vi "WVD Calculation.vi"(1 "time increment":i32, 2 "H[s]":dbl[](array[numeric]) format="%.2f", 3 "s":dbl[](array[numeric]) format="%.2f") -> (0 "Fourier[s(i-m)*g(m)]":sgl[][](array[numeric]) format="%.2f")   [LabVIEW 2017, in "NI_Gmath.lvlib"]
uses:
  <vilib>/gmath/NI_Gmath.lvlib
  <vilib>/Analysis/2dsp.llb/Complex FFT.vi
  <vilib>/Analysis/NI_AALPro.lvlib
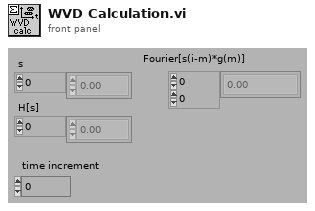
[diagram p1: front panel]
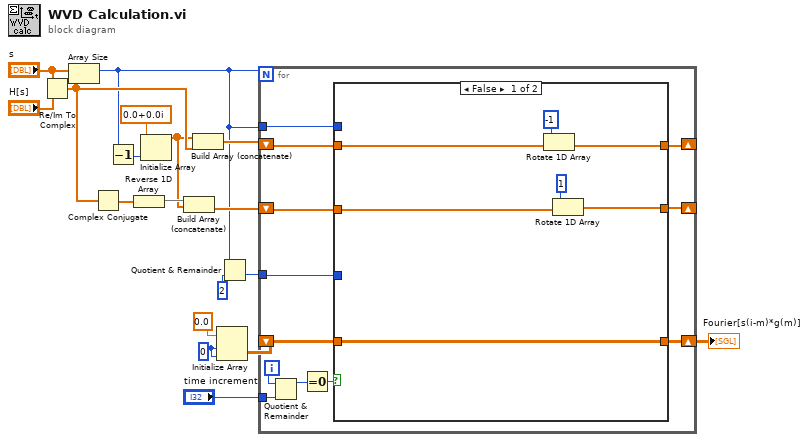
[diagram p0: block diagram]
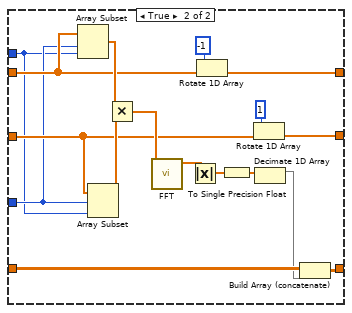
[diagram p2: hidden frame]
diagram:
  w1 = 0
  n1 = Re/Im To Complex(1:"H[s]", 2:"s") -> (0:w12:cdb[])
  n2 = Array Size(array="s") -> (size(s)=w6:i32)
  n3 = Complex Conjugate(1:w12) -> (0:w11:cdb[])
  n4 = Decrement(x=w6) -> (x-1=w18:i32)
  n5 = Reverse 1D Array(array=w11) -> (reversed array=w15:cdb[])
  n6 = Initialize Array(csg 0.0+0.0i, w18) -> (w8:csg[])
  n7 = Build Array (concatenate)(w15, w8) -> (w14:cdb[])
  n8 = Build Array (concatenate)(w8, w12) -> (w16:cdb[])
  n9 = Initialize Array(sgl 0.0, w1, w1) -> (w4:sgl[][])
  n10 = Quotient & Remainder(x=w6, y=2) -> (floor(x/y)=w9:i32)  [unwired: 1 out]
  n11 = for {
    N: w6 -> [_]
    shift-right: [w30] -> _
    shift-left: w16 -> [w26]
    shift-right: [w29] -> _
    shift-left: w14 -> [w25]
    tunnel: w6 -> [w28]
    tunnel: w9 -> [w27]
    shift-right: [w19] -> w2
    shift-left: w4 -> [w20]
    tunnel: "time increment" -> [w23]
    i -> [w24]
    n12 = Quotient & Remainder(x=w24, y=w23) -> (x-y*floor(x/y)=w22:i32)  [unwired: 1 out]
    n13 = Equal To 0?(x=w22) -> (x = 0?=w21:bool)
    n14 = case shown="False" w21 {
      tunnel: w25 -> [w32 w49]
      tunnel: w26 -> [w34 w47]
      tunnel: w27 -> [_ w46]
      tunnel: w28 -> [_ w45]
      tunnel: [w31 w44] -> w29
      tunnel: [w33 w41] -> w30
      tunnel: w20 -> [w37 w40]
      tunnel: [w37 w39] -> w19
      frame False {
        n15 = Rotate 1D Array(1:w34, 2:-1) -> (0:w33:cdb[])
        n16 = Rotate 1D Array(1:w32, 2:1) -> (0:w31:cdb[])
      }
      frame True {
        n17 = Array Subset(array=w47, index=w46, length=w45) -> (w48:cdb[])
        n18 = Array Subset(array=w49, index=w46, length=w45) -> (w50:cdb[])
        n19 = Multiply(x=w48, y=w50) -> (x*y=w51:cdb[])
        n20 = call-poly <vilib>:"FFT.vi"("X"=w51) -> ("FFT {X}"=w52:cdb[])  [unwired: 9 in, 1 out]
        n21 = Absolute Value(x=w52) -> (abs(x)=w53:dbl[])
        n22 = Rotate 1D Array(1:w47, 2:-1) -> (0:w41:cdb[])
        n23 = To Single Precision Float(number=w53) -> (single precision float=w54:sgl[])
        n24 = Rotate 1D Array(1:w49, 2:1) -> (0:w44:cdb[])
        n25 = Decimate 1D Array(w54) -> (w38:sgl[])  [unwired: 1 out]
        n26 = Build Array (concatenate)(w40, w38) -> (w39:sgl[][])
      }
    }
  }
  "Fourier[s(i-m)*g(m)]" <- w2
